vi "Untitled 1.vi"() -> ()   [LabVIEW 2010]
panel:
  out "unsigned 32bit integer":u32
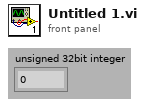
[diagram p1: front panel]
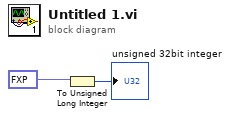
[diagram p0: block diagram]
diagram:
  n1 = To Unsigned Long Integer(number=fxp<+/-,8,10> -500.0) -> (unsigned 32bit integer=→"unsigned 32bit integer":u32)
